vi "Subscriber2.vi"() -> ()   [LabVIEW 2021]
uses:
  ChannelCommon/typedef/Datatype Waveform.ctl
  CIFChannels/Typedef/Direction.ctl
  ChannelCommon/typedef/FIFO Config.ctl
  CIF_NIChn/FIFO_DAQ/CIF_NIChn_Fifo_DAQ.lvclass
  D:/dev/Packages/Channel_Manager/src/CIFChannels/CIFChannels.lvclass
  D:/dev/Packages/Channel_Manager/src/CIF_NIChn/NIChn/CIF_NIChn.lvclass
  CIFChannels/CIFChannels.lvclass/CIFChannels.ctl
  CIF_NIChn/NIChn/CIF_NIChn.lvclass/CIF_NIChn.ctl
  CIF_NIChn/FIFO_DAQ/CIF_NIChn_Fifo_DAQ.lvclass/CIF_NIChn_Fifo_DAQ.ctl
  <vilib>/CIF Foundation/CIF Utilities/Statistics/I64/Stats_I64_CIF_U.lvclass/Stats_I64_CIF_U.ctl
  <vilib>/CIF Foundation/CIF Utilities/DataTypes/Flatten U64.vi
  CIF_NIChn/FIFO_DAQ/SubVIs/Core Read DAQ FIFO.vi
  CIF_NIChn/FIFO_DAQ/SubVIs/Core Read DAQ FIFO.vi/a66d495f-c29f-4596-8ad9-13e7f334244d.vi
  CIF_NIChn/FIFO_DAQ/SubVIs/Core Read DAQ FIFO.vi/010c5156-5ad7-4e56-b6b0-a69033aca011.vi
  CIFChannels/Utilities/Update Flatten Benchmark.vi
  CIF_NIChn/FIFO_DAQ/SubVIs/Core Read DAQ DVR FIFO.vi
  <vilib>/CIF Foundation/CIF Utilities/Time/System Time/Get System Time.vi
  <vilib>/CIF Foundation/CIF Utilities/Statistics/I64/X1 minus X0.vi
  CIF_NIChn/NIChn/Accessors/Read CIF Channel.vi
  CIF_NIChn/NIChn/SubVIs/Check Disconnect.vi
  <vilib>/CIF Foundation/CIF Channels/CIFChannels/Top Level/Read U8 Array.vi
  ChannelCommon/Utilities/Unflatten Header.vi
  CIFChannels/Utilities/Update Channel Benchmark.vi
  CIF_NIChn/FIFO_DAQ/SubVIs/Core Read DAQ DVR FIFO.vi/683dda70-af16-44bc-a524-9971cb6dbe1c.vi
  CIF_NIChn/FIFO_DAQ/SubVIs/Core Read DAQ DVR FIFO.vi/9ab161bc-d75a-4f10-a981-8d657be3a6b1.vi
  CIFChannels/Accessors/Read Channel State.vi
  CIFChannels/Accessors/Read Direction.vi
  CIF_NIChn/FIFO_DAQ/SubVIs/Unflatten.vi
  <vilib>/CIF Foundation/CIF Utilities/Time/System Time/LabVIEW Time to TAI Time.vi
  <vilib>/CIF Foundation/CIF Utilities/Statistics/I64/X1 minus X0.vi/dfabcf33-0dbc-4041-80a5-3dc0c86d2989.vi
  CIFChannels/Accessors/Write Channel State.vi
  CIFChannels/Accessors/Read Tag Disconnect Behavior.vi
  <vilib>/CIF Foundation/CIF Channels/CIFChannels/Top Level/Read U8 Array.vi/4bc1c15b-36ab-481f-b8dd-c64075ce723a.vi
  <vilib>/CIF Foundation/CIF Channels/CIFChannels/Top Level/Read U8 Array.vi/d83cb72b-7713-41fc-a3d1-682de79cf574.vi
  <vilib>/CIF Foundation/CIF Channels/CIFChannels/SubVIs/Get dll Path.vi
  <vilib>/CIF Foundation/CIF Channels/CIFChannels/SubVIs/Get Requested Size.vi
  <vilib>/CIF Foundation/CIF Utilities/DataTypes/Unflatten U64.vi
  <vilib>/CIF Foundation/CIF Utilities/DataTypes/Unflatten I64.vi
  ChannelCommon/Utilities/Add Error.vi
  ChannelCommon/CIFFIFO/Flatten/DVR Unflatten.vi
  CIFChannels/Accessors/Write FIFO Header.vi
  CIFChannels/Accessors/Write FIFO Timeout.vi
  <vilib>/CIF Foundation/CIF Utilities/Statistics/I64/X1 minus X0.vi/dfabcf33-0dbc-4041-80a5-3dc0c86d2989.vi/9eb60a9a-770f-4d2d-8b3f-8465c267ecc9.vi
  <vilib>/CIF Foundation/CIF Utilities/Errors/Append Error Location.vi
  CIF_NIChn/NIChn/CIF_NIChn.lvclass
  ChannelCommon/ChannelCommon.lvlib
  CIFChannels/CIFChannels.lvclass
panel:
  out "DAQ Out":T1[](array[typedef])
  in  "stop":bool
  in  "Publisher":string
  out "pass":bool
  out "error out":errorcluster
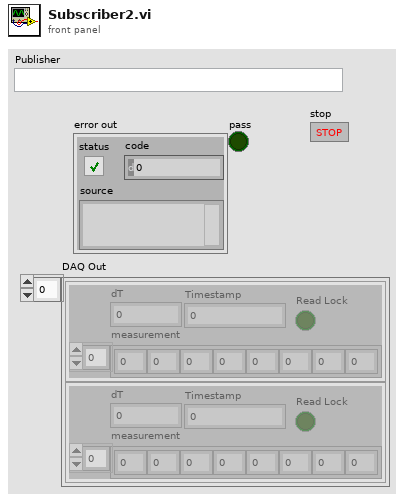
[diagram p1: front panel]
types:
  T1 = typedef "ChannelCommon.lvlib/Datatype Waveform.ctl" = cluster{"measurement":dbl[], "dT":dbl, "Timestamp":i64, "Read Lock":bool}
  T2 = typedef "ChannelCommon.lvlib/FIFO Config.ctl" = cluster{"Max Bytes/Msg":u64, "Max Msg/FIFO":u64, "Flags":u64}
  T3 = typedef "CIFChannels.lvclass/Direction.ctl" = enum16{"Publisher", "Subscriber"}
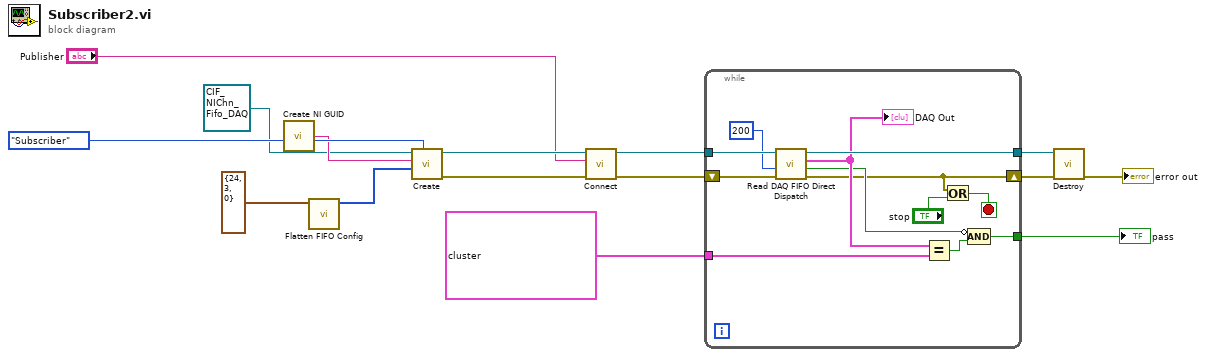
[diagram p0: block diagram]
diagram:
  n1 = call <vilib>:"Create NI GUID.vi"() -> ("NI GUID"=w12:string)
  n2 = call "Flatten FIFO Config.vi"("FIFO Config in"=T2 {"Max Bytes/Msg"=24, "Max Msg/FIFO"=3, "Flags"=0}) -> ("Flattened FIFO Config"=w6:u8[])  [unwired: 10 in]
  n3 = call-dynamic "Create.vi"("Direction"=Direction."Subscriber", "Custom Config Data"=w6, "Name"=w12, "CIFTag in"=refnum<class "CIF_NIChn_Fifo_DAQ.lvclass"> refnum ("CIF_NIChn_Fifo_Power.lvclass")) -> ("error out"=w10:errorcluster, "CIFTag out"=w9:refnum<class "CIF_NIChn_Fifo_DAQ.lvclass">)  [unwired: 6 in]
  n4 = call-dynamic "Connect.vi"("error in (no error)"=w10, "Connection Name"="Publisher", "CIFTag in"=w9) -> ("error out"=w2:errorcluster, "CIFTag out"=w8:refnum<class "CIF_NIChn_Fifo_DAQ.lvclass">)  [unwired: 7 in]
  n5 = while {
    tunnel: [w27] -> w14
    tunnel: w8 -> [w25]
    tunnel: T1[] [{"measurement"=array[986 elements], "dT"=43.0, "Timestamp"=2, "Read Lock"=FALSE}, {"measurement"=array[1001 elements], "dT"=34.0, "Timestamp"=1, "Read Lock"=FALSE}] ("DAQ In") -> [w21]
    tunnel: [w20] -> w5
    shift-right: [w18] -> w1
    shift-left: w2 -> [w19]
    stop <- w16 stop-if-true
    n6 = call "Read DAQ FIFO Direct Dispatch.vi"("error in (no error)"=w19, "Timeout (ms)"=200, "CIFTag in"=w25) -> ("error out"=w18:errorcluster, "timed out?"=w23:bool, "DAQ Out"=w24:T1[], "CIFTag out"=w27:refnum<class "CIF_NIChn_Fifo_DAQ.lvclass">)  [unwired: 4 in, 1 out]
    "DAQ Out" <- w24
    n7 = Equal?(x=w24, y=w21) -> (x = y?=w26:bool)
    n8 = Or(x=w18, y="stop") -> (x .or. y?=w16:bool)
    n9 = Compound Arithmetic op=AND(invert w23, w26) -> (w20:bool)
  }
  "pass" <- w5
  n10 = call-dynamic "Destroy.vi"("error in (no error)"=w1, "CIF_NIChn_Fifo_Power_DVR in"=w14) -> ("error out"=→"error out":errorcluster)  [unwired: 8 in, 1 out]
